vi "DateShift.vi"() -> (0 "RealTime":string, 1 "NameTime":string, 2 "DateShift":string)   [LabVIEW 2017]
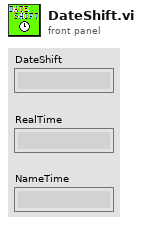
[diagram p1: front panel]
types:
  T1 = typedef "LVDateTimeRec.ctl" = cluster{"fractional second":dbl, "second":i32, "minute":i32, "hour":i32, "day of month":i32, "month":i32, "year":i32, "day of week":i32, "day of year":i32, "DST":i32}
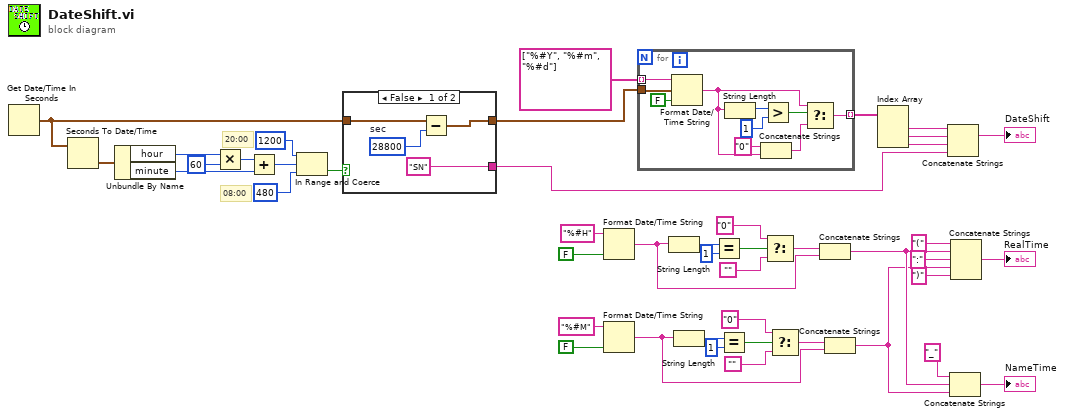
[diagram p0: block diagram]
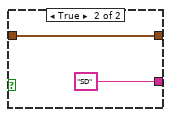
[diagram p2: hidden frame]
diagram:
  # "08:00"
  # "20:00"
  n1 = Get Date/Time In Seconds() -> (seconds since 1Jan1904=w44:timestamp)
  n2 = Seconds To Date/Time(time stamp (now)=w44) -> (date time rec=w43:T1)  [unwired: 1 in]
  n3 = Unbundle By Name(w43) -> ("hour"=w40:i32, "minute"=w39:i32)
  n4 = Multiply(x=w40, y=60) -> (x*y=w41:i32)
  n5 = Add(x=w41, y=w39) -> (x+y=w38:i32)
  n6 = In Range and Coerce(upper limit=1200 ("y"), x=w38, lower limit=480 ("y")) -> (In Range?=w35:bool)  [unwired: 1 out]
  n7 = case shown="False" w35 {
    tunnel: w44 -> [w47 w50]
    tunnel: [w46 w50] -> w33
    tunnel: ["SN" "SD"] -> w27
    frame False {
      w48 = 28800  # sec
      n8 = Subtract(x=w47, y=w48) -> (x-y=w46:timestamp)
    }
    frame True {
    }
  }
  n9 = Format Date/Time String(time format string (%c)="%#H", UTC format=FALSE) -> (date/time string=w16:string)  [unwired: 1 in]
  n10 = Format Date/Time String(time format string (%c)="%#M", UTC format=FALSE) -> (date/time string=w9:string)  [unwired: 1 in]
  n11 = for {
    tunnel: string[] ["%#Y", "%#m", "%#d"] -> [w60] mode=indexing
    tunnel: w33 -> [w58]
    tunnel: [w54] -> w32 mode=indexing
    n12 = Format Date/Time String(time format string (%c)=w60, seconds (now)=w58, UTC format=FALSE) -> (date/time string=w56:string)
    n13 = String Length(string=w56) -> (length=w52:i32)
    n14 = Concatenate Strings("0" ("string"), w56) -> (w55:string)
    n15 = Greater?(x=w52, y=1) -> (0:w53:bool)
    n16 = Select(t=w56, s=w53, f=w55) -> (s? t:f=w54:string)
  }
  n17 = String Length(string=w16) -> (length=w22:i32)
  n18 = String Length(string=w9) -> (length=w10:i32)
  n19 = Equal?(x=w22, y=1) -> (x = y?=w20:bool)
  n20 = Equal?(x=w10, y=1) -> (x = y?=w12:bool)
  n21 = Select(t="0", s=w20, f="") -> (s? t:f=w17:string)
  n22 = Select(t="0", s=w12, f="") -> (s? t:f=w15:string)
  n23 = Concatenate Strings(w17, w16) -> (w3:string)
  n24 = Concatenate Strings(w15, w9) -> (w2:string)
  n25 = Index Array(array=w32) -> (element #1=w31:string, element #2=w30:string, element #3=w29:string)  [unwired: 3 in]
  n26 = Concatenate Strings(w31, w30, w29, w27) -> (→"DateShift":string)
  n27 = Concatenate Strings("_" ("string"), w3, w2) -> (→"NameTime":string)
  n28 = Concatenate Strings("(" ("string"), w3, ":" ("string"), w2, ")" ("string")) -> (→"RealTime":string)
